vi "Init4118.vi"(6 "Temperature":refnum<vi>, 8 "error in (no error)":errorcluster, 9 "FetchData":T1, 10 "ThermocoupleSetting":T2={"Interface"="", "value range"="T/C T type -100 ~ 400 degree C", "Channel Count"=8, "Limit 0"=0.0, "Limit 1"=0.0, "Limit 2"=0.0, "Limit 3"=0.0, "Limit 4"=0.0, "Limit 5"=0.0, "Limit 6"=0.0, "Limit 7"=0.0} caption="Thermocouple" {"Limit 7" format="%.1f"; "Limit 6" format="%.1f"; "Limit 5" format="%.1f"; "Limit 4" format="%.1f"; "Limit 3" format="%.1f"; "Limit 2" format="%.1f"; "Limit 1" format="%.1f"; "Limit 0" format="%.1f"; "Channel Count" min=0 max=24}, 11 "4118 in":refnum<class "4118.lvclass">) -> (0 "error out":errorcluster, 3 "4118 out":refnum<class "4118.lvclass">)   [LabVIEW 2024, in "4118 Actor.lvlib" / "4118.lvclass"]
uses:
  4118.lvclass
  4118.lvclass/4118.ctl
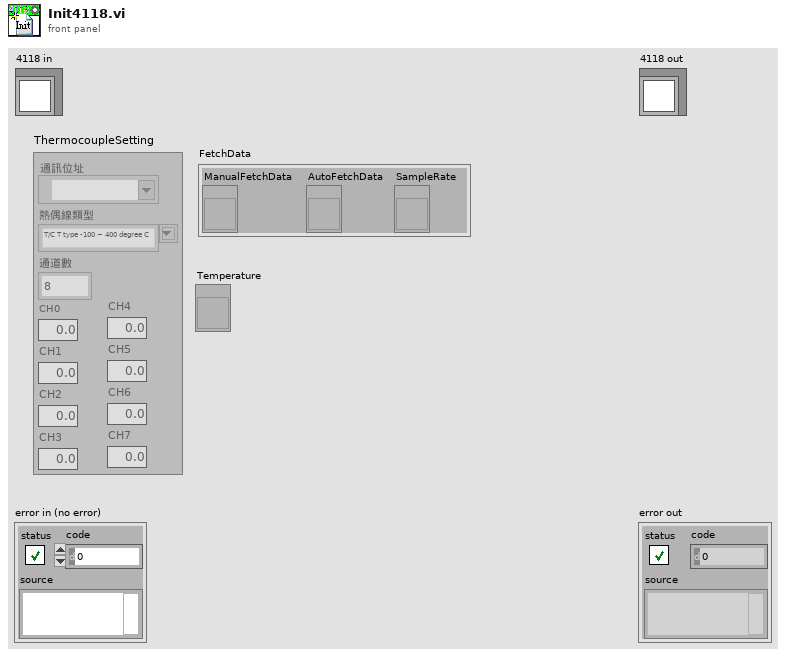
[diagram p1: front panel]
types:
  T1 = cluster{"ManualFetchData":refnum<vi>, "AutoFetchData":refnum<vi>, "SampleRate":refnum<vi>}
  T2 = cluster{"Interface":refnum<visa-resource-name>, "value range":string, "Channel Count":i32, "Limit 0":dbl, "Limit 1":dbl, "Limit 2":dbl, "Limit 3":dbl, "Limit 4":dbl, "Limit 5":dbl, "Limit 6":dbl, "Limit 7":dbl}
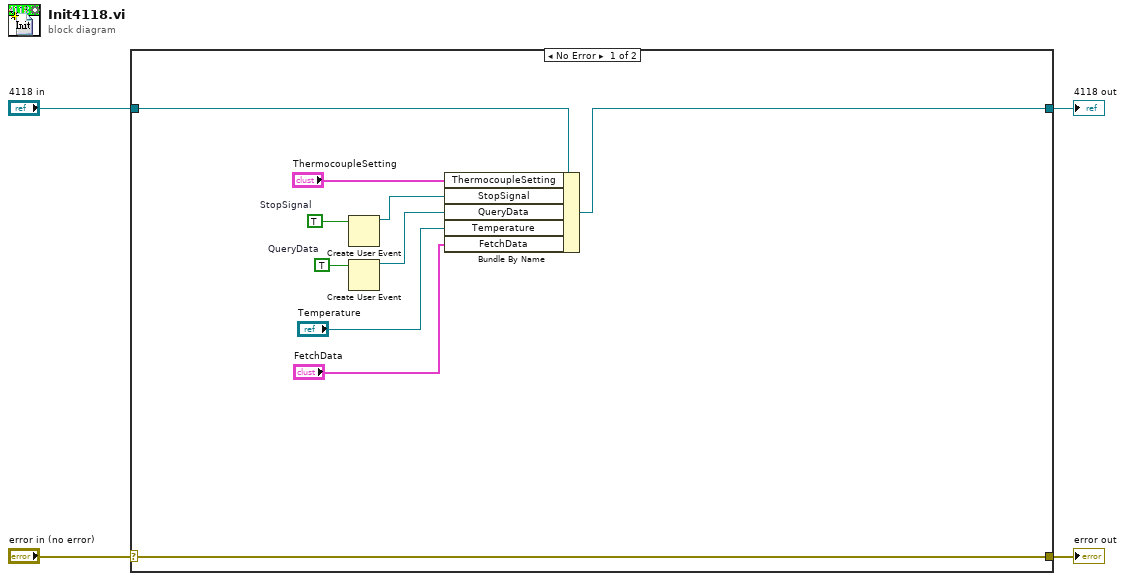
[diagram p0: block diagram]
diagram:
  n1 = case shown="No Error" "error in (no error)" {
    selector: "error in (no error)" -> [w14 w16]
    tunnel: [w14 w16] -> w3
    tunnel: [w5 w15] -> w1
    tunnel: "4118 in" -> [w13 w15]
    frame No Error {
      w9 = TRUE  # QueryData
      w11 = TRUE  # StopSignal
      n2 = Create User Event(user event datatype=w11) -> (user event=w10:refnum<user-event>)  [unwired: 1 in, 1 out]
      n3 = Create User Event(user event datatype=w9) -> (user event=w8:refnum<user-event>)  [unwired: 1 in, 1 out]
      n4 = Bundle By Name(cluster=w13, "ThermocoupleSetting"="ThermocoupleSetting", "StopSignal"=w10, "QueryData"=w8, "Temperature"="Temperature", "FetchData"="FetchData") -> (w5:refnum<class "4118.lvclass">)
    }
    frame Error {
    }
  }
  "error out" <- w3
  "4118 out" <- w1
